vi "Create.vi"(8 "error in (no error)":errorcluster, 10 "New Client Q":refnum<queue>) -> (0 "error out":errorcluster, 3 "SSE Manager out":refnum<class "SSE Manager.lvclass">)   [LabVIEW 2020, in "Server Sent Events Example.lvlib" / "SSE Manager.lvclass"]
uses:
  SSE Manager.lvclass
  SSE Manager.lvclass/SSE Manager.ctl
  lv-http-server/HTTP Server/SSE Client/SSE Client.lvclass
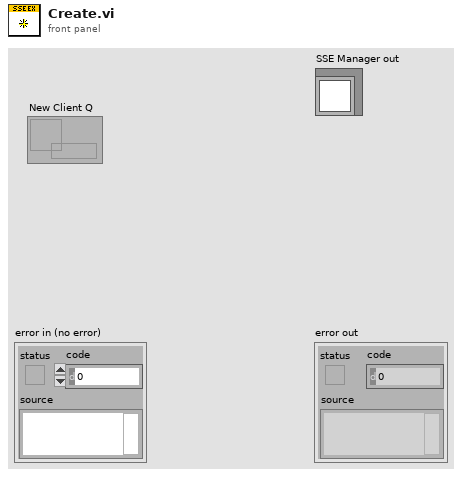
[diagram p1: front panel]
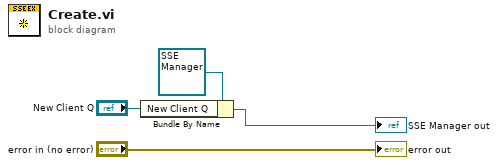
[diagram p0: block diagram]
diagram:
  n1 = Bundle By Name(cluster=refnum<class "SSE Manager.lvclass"> refnum ("SSE Manager in"), "New Client Q"="New Client Q") -> (→"SSE Manager out":refnum<class "SSE Manager.lvclass">)
  "error out" <- "error in (no error)"
